vi "KE622x -- Set Triax Inner Shield Connection.vi"(0 "Resource In":refnum<visa-resource-name>, 1 "Check For SCPI Errors? (T)":bool=TRUE, 7 "Triax Inner Shield Connection":T1=enum."Cable Guard", 11 "error in (no error)":errorcluster) -> (4 "Resource Out (dupl)":refnum<visa-resource-name>, 15 "error out":errorcluster)   [LabVIEW 2019, in "Keithley 622x.lvlib"]
doc: "Controls where the inner shield of the triax output is connected to, either 'Output Low' (the current source's low output) or 'Cable Guard'. Note that setting the inner triax connection _does not_ affect the low output connection set via 'KE622x -- Set Output Low Connection'. Essentially, the low output can connected to either 'Earth Ground' (low output connected to outer shield of triax connector) or 'Floating' (low output connected to rear panel LO banana jack), _independently_ of whether or not the inner triax shield is connected to it as well."
uses:
  Keithley 622x.lvlib
  Typedefs/KE622x -- Triax Inner Shield Connection.ctl
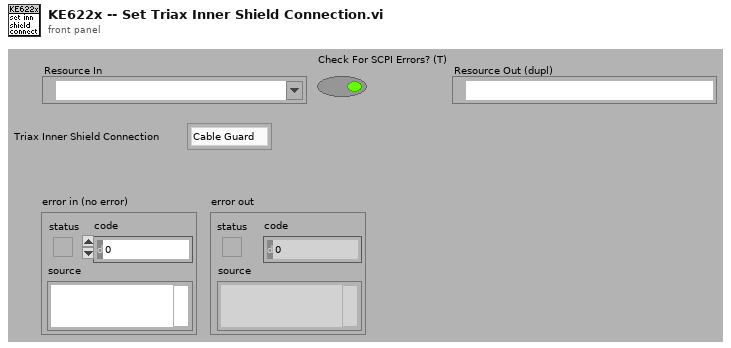
[diagram p1: front panel]
types:
  T1 = typedef "Keithley 622x.lvlib/KE622x -- Triax Inner Shield Connection.ctl" = enum16{"Output Low", "Cable Guard"}
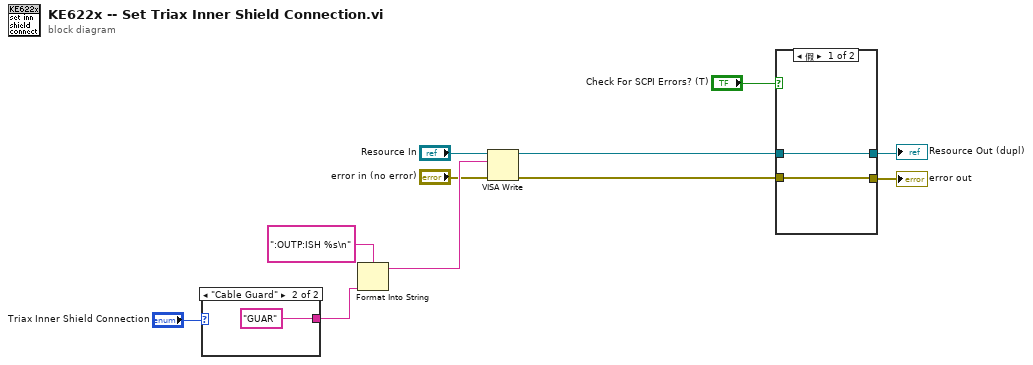
[diagram p0: block diagram]
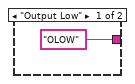
[diagram p2: hidden frame]
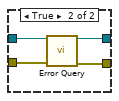
[diagram p3: hidden frame]
diagram:
  n1 = case shown="\"Cable Guard\"" "Triax Inner Shield Connection" {
    tunnel: ["OLOW" "GUAR"] -> w1
    frame "Output Low" {
    }
    frame "Cable Guard" {
    }
  }
  n2 = Format Into String(format string=":OUTP:ISH %s\n", w1) -> (resulting string=w9:string)  [unwired: 2 in, 1 out]
  n3 = VISA Write(VISA resource name="Resource In", write buffer=w9, error in (no error)="error in (no error)") -> (VISA resource name out=w6:refnum<visa-resource-name>, error out=w5:errorcluster)  [unwired: 1 out]
  n4 = case shown="假" "Check For SCPI Errors? (T)" {
    tunnel: w6 -> [w15 w19]
    tunnel: w5 -> [w14 w18]
    tunnel: [w14 w17] -> w3
    tunnel: [w15 w16] -> w4
    frame False {
    }
    frame True {
      n5 = call "Error Query.vi"("VISA Resource In"=w19, "error in (no error)"=w18) -> ("VISA Resource Out (dupl)"=w16:refnum<visa-resource-name>, "error out"=w17:errorcluster)  [unwired: 10 in, 2 out]
    }
  }
  "Resource Out (dupl)" <- w4
  "error out" <- w3
